vi "Software Watchdog.vi"(8 "Timeout":i32, 10 "Wack":bool, 11 "Run":bool) -> (0 "Running":bool, 2 "Count":i32, 3 "Expired":bool)   [LabVIEW 2011]
panel:
  out "Wacked":bool
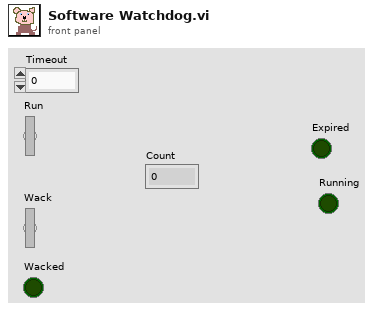
[diagram p1: front panel]
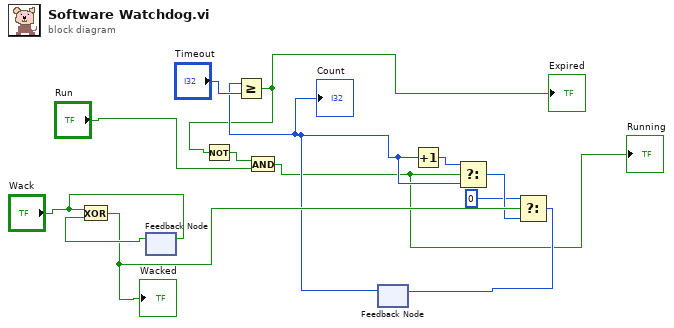
[diagram p0: block diagram]
diagram:
  n1 = feedback-in #1("Wack") -> ()
  n2 = feedback #1() -> (w11:bool)  [unwired: 1 in]
  n3 = Exclusive Or(1:w11, 2:"Wack") -> (0:w9:bool)
  "Wacked" <- w9
  n4 = feedback #2() -> (w5:i32)  [unwired: 1 in]
  "Count" <- w5
  n5 = Greater Or Equal?(x=w5, y="Timeout") -> (x >= y?=w1:bool)
  "Expired" <- w1
  n6 = Not(x=w1) -> (.not. x?=w2:bool)
  n7 = And(x=w2, y="Run") -> (x .and. y?=w3:bool)
  "Running" <- w3
  n8 = Increment(x=w5) -> (x+1=w13:i32)
  n9 = Select(t=w13, s=w3, f=w5) -> (s? t:f=w8:i32)
  n10 = Select(t=0, s=w9, f=w8) -> (s? t:f=w10:i32)
  n11 = feedback-in #2(w10) -> ()
